vi "Send Message.vi"(6 "Message Priority":enum16{"Normal", "High"}(ring), 8 "error in":errorcluster, 10 "Message Payload in":refnum<class "IMessagePayload.lvclass">, 11 "QueueMessageTransport in":refnum<class "QueueMessageTransport.lvclass">) -> (0 "error out":errorcluster, 3 "QueueMessageTransport out":refnum<class "QueueMessageTransport.lvclass">)   [LabVIEW 2016, in "QueueMessageTransport.lvclass"]
uses:
  QueueMessageTransport.lvclass
  IMessagePayload/IMessagePayload.lvclass
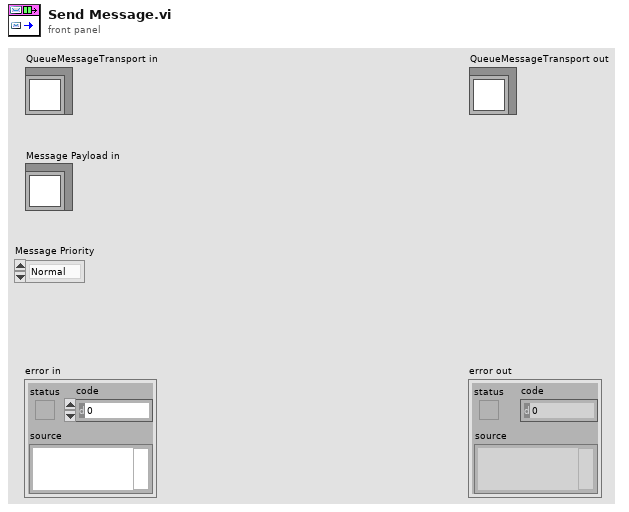
[diagram p1: front panel]
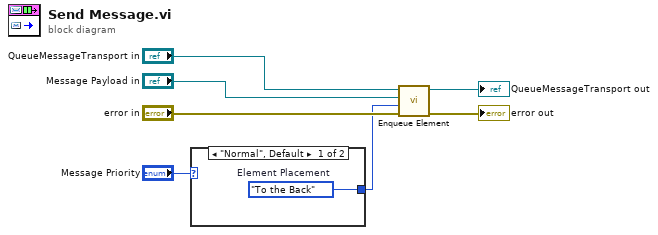
[diagram p0: block diagram]
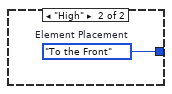
[diagram p2: hidden frame]
diagram:
  n1 = case shown="\"Normal\", Default" "Message Priority" {
    tunnel: [w8 w9] -> w1
    frame "Normal", Default {
      w8 = enum16{"To the Front", "To the Back"}."To the Back"  # Element Placement
    }
    frame "High" {
      w9 = enum16{"To the Front", "To the Back"}."To the Front"  # Element Placement
    }
  }
  n2 = call "Enqueue Element.vi"("error in"="error in", "Element Placement"=w1, "Q Element"="Message Payload in", "QueueMessageTransport in"="QueueMessageTransport in") -> ("error out"=→"error out":errorcluster, "QueueMessageTransport out"=→"QueueMessageTransport out":refnum<class "QueueMessageTransport.lvclass">)  [unwired: 6 in]
